vi "DaqOscilloscope.vi"() -> ()   [LabVIEW 2025]
panel:
  out "Waveform Graph":waveform(dbl)[](graph)
  out "error out":errorcluster
  in  "physical channels":tag
  in  "channel settings":T1={"units"=10348, "input terminal configuration"=-1, "maximum value"=5.0, "minimum value"=-5.0} {"units" items=["Volts"=10348, "From Custom Scale"=10065]; "input terminal configuration" items=["Default"=-1, "RSE"=10083, "NRSE"=10078, "Differential"=10106, "Pseudodifferential"=12529]}
  in  "frequency settings":T2={"frequency (Hz)"=0.001, "number of samples per cycle"=2.0, "number of cycles"=1.0} {"frequency (Hz)" min=0.001 max=100000000.0; "number of samples per cycle" min=2.0 step=1.0; "number of cycles" min=1.0}
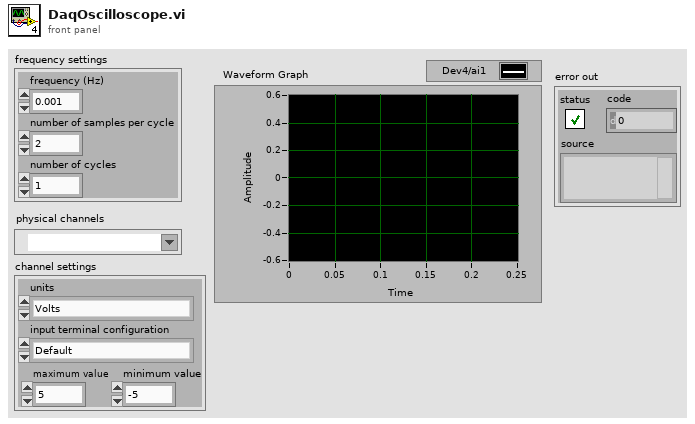
[diagram p1: front panel]
types:
  T1 = cluster{"units":i32, "input terminal configuration":i32, "maximum value":dbl, "minimum value":dbl}
  T2 = cluster{"frequency (Hz)":dbl, "number of samples per cycle":dbl, "number of cycles":dbl}
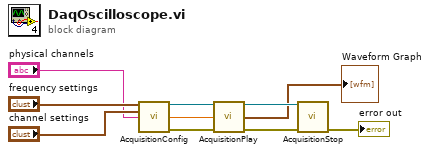
[diagram p0: block diagram]
diagram:
  n1 = call "AcquisitionConfig.vi"("frequency settings"="frequency settings", "channel settings"="channel settings", "physical channels"="physical channels") -> ("task out"=w10:refnum<k21>, "number of samples"=w1:dbl, "error out"=w2:errorcluster)  [unwired: 10 in]
  n2 = call "AcquisitionPlay.vi"("task/channels in"=w10, "number of samples per channel"=w1, "error in"=w2) -> ("task out"=w9:refnum<k21>, "data"=→"Waveform Graph":waveform(dbl)[], "error out"=w8:errorcluster)  [unwired: 10 in]
  n3 = call "AcquisitionStop.vi"("task/channels in"=w9, "error in"=w8) -> ("error out"=→"error out":errorcluster)  [unwired: 13 in]
